vi "FPGAController_v3.vi"() -> ()   [LabVIEW 2012]
uses:
  <vilib>/Utility/miscctls.llb/LVPointTypeDef.ctl
  Functional Global Variables/Action Items.ctl
  <vilib>/FPGAPlugInAG/PXI-7954R/niLvFpga_Open_PXI-7954R.vi
  <vilib>/addons/database/Connection.llb/Conn Execute.vi
  <vilib>/addons/database/Recordset.llb/Rec Fetch Recordset Data (R).vi
  <vilib>/addons/database/Recordset.llb/Rec Destroy - Connection.vi
  <vilib>/Utility/error.llb/Error Cluster From Error Code.vi
  <vilib>/rvi/errors/niLvFpgaAdjustHostInterfaceError.vi
  <vilib>/FPGAPlugInAG/PXI-7954R/niLvFpga_Close_PXI-7954R.vi
  <vilib>/rvi/interface/nirviOpenFPGA/nirviOpenFPGA.xnode
  FPGA Bitfiles/correlationwithf_FPGATarget_ver1(FPGA)214201_xVEwbWkwy+w.lvbitx
  ver1(FPGA)_7_8_2013.vi
  <vilib>/rvi/interface/nirviMethod/nirviMethod.xnode
  <vilib>/FPGA/interface/niFpgaViExecutionMode.ctl
  <vilib>/addons/database/_DB Variant To Data/Database Variant To Data.xnode
  <vilib>/rvi/interface/nirviReadWriteControl/nirviReadWriteControl.xnode
  FPGA Bitfiles/correlationwithf_FPGATarget_ver1(FPGA)214201_RJg2enFNf9w.lvbitx
  <vilib>/rvi/interface/nirviCloseFPGA/nirviCloseFPGA.xnode
  <vilib>/addons/database/NI_Database_API.lvlib
  NiFpgaLv.dll
  <vilib>/FPGAPlugInAG/PXI-7954R/niLvFpga_Reset_PXI-7954R.vi
  <vilib>/FPGAPlugInAG/PXI-7954R/niLvFpga_Run_PXI-7954R.vi
panel:
  out "Rearm Trigger":bool
  in  "Rearm Trigger":bool
  in  "One Shot Mode":bool
  out "Last Update:":timestamp
  out "Updating FPGA":bool
  out "Sensitivity":dbl
  out "error out":errorcluster
  out "Low Mass Limit":fxp<+,31,17>
  out "High Mass Limit":fxp<+,31,17>
  out "stopping":bool
  in  "Auto Threshold":bool
  out "Peletron (MV)":dbl=2.0
  out "High Mass (kg)":dbl=inf
  out "Low Mass (kg)":dbl
  out "High Charge Limit":i16
  out "Low Charge Limit":i16
  out "High velocity count":i32=210
  out "Low velocity count":i32=21000
  in  "stop":bool
  in  "Peak-Threshold Factor":dbl=3.0
  out "Low Charge Limit (fC)":dbl
  out "High Charge Limit (fC)":dbl=100.0
  out "High Velocity":dbl=100000.0
  out "Low Velocity":dbl=1000.0
  out "Filter 7 Peak":i32=7483
  out "Filter 6 Peak":i32=9863
  out "Filter 5 Peak":i32=13910
  out "Filter 4 Peak":i32=18191
  out "Filter 3 Peak":i32=46254
  out "Filter 2 Peak":i32=120664
  out "Filter 1 Peak":i32=295996
  in  "Filter7 Threshold":i32=-21165
  in  "Filter6 Threshold":i32=-29358
  in  "Filter5 Threshold":i32=-41730
  in  "Filter4 Threshold":i32=-54306
  in  "Filter3 Threshold":i32=-138762
  in  "Filter2 Threshold":i32=-361992
  in  "Filter1 Threshold":i32=-887988
  in  "Zero Peak Values":bool
  in  "Assign Threshold":bool
  in  "Run Mode":bool
  # "Settings"
  # "Dubugging"
  # "Independent Variable"
  # "Low Vel."
  # "High Vel."
  # "Low Q (fC)"
  # "High Q (fC)"
  # "Plate Control While Loop Counter"
  # "Low Mass (kg)"
  # "High Mass (kg)"
  # "Sens. (V/pC)"
  # "Peletron (MV)"
  # "Current Value of Running Average"
  # "Peak Threshold Factor"
  # "Peak Values"
  # "Peak 1"
  # "Peak 2"
  # "Peak 3"
  # "Peak 4"
  # "Peak 5"
  # "Peak 6"
  # "Peak 7"
  # "Thresholds"
  # "Threshold 1"
  # "Threshold 2"
  # "Threshold 3"
  # "Threshold 4"
  # "Threshold 5"
  # "Threshold 6"
  # "Threshold 7"
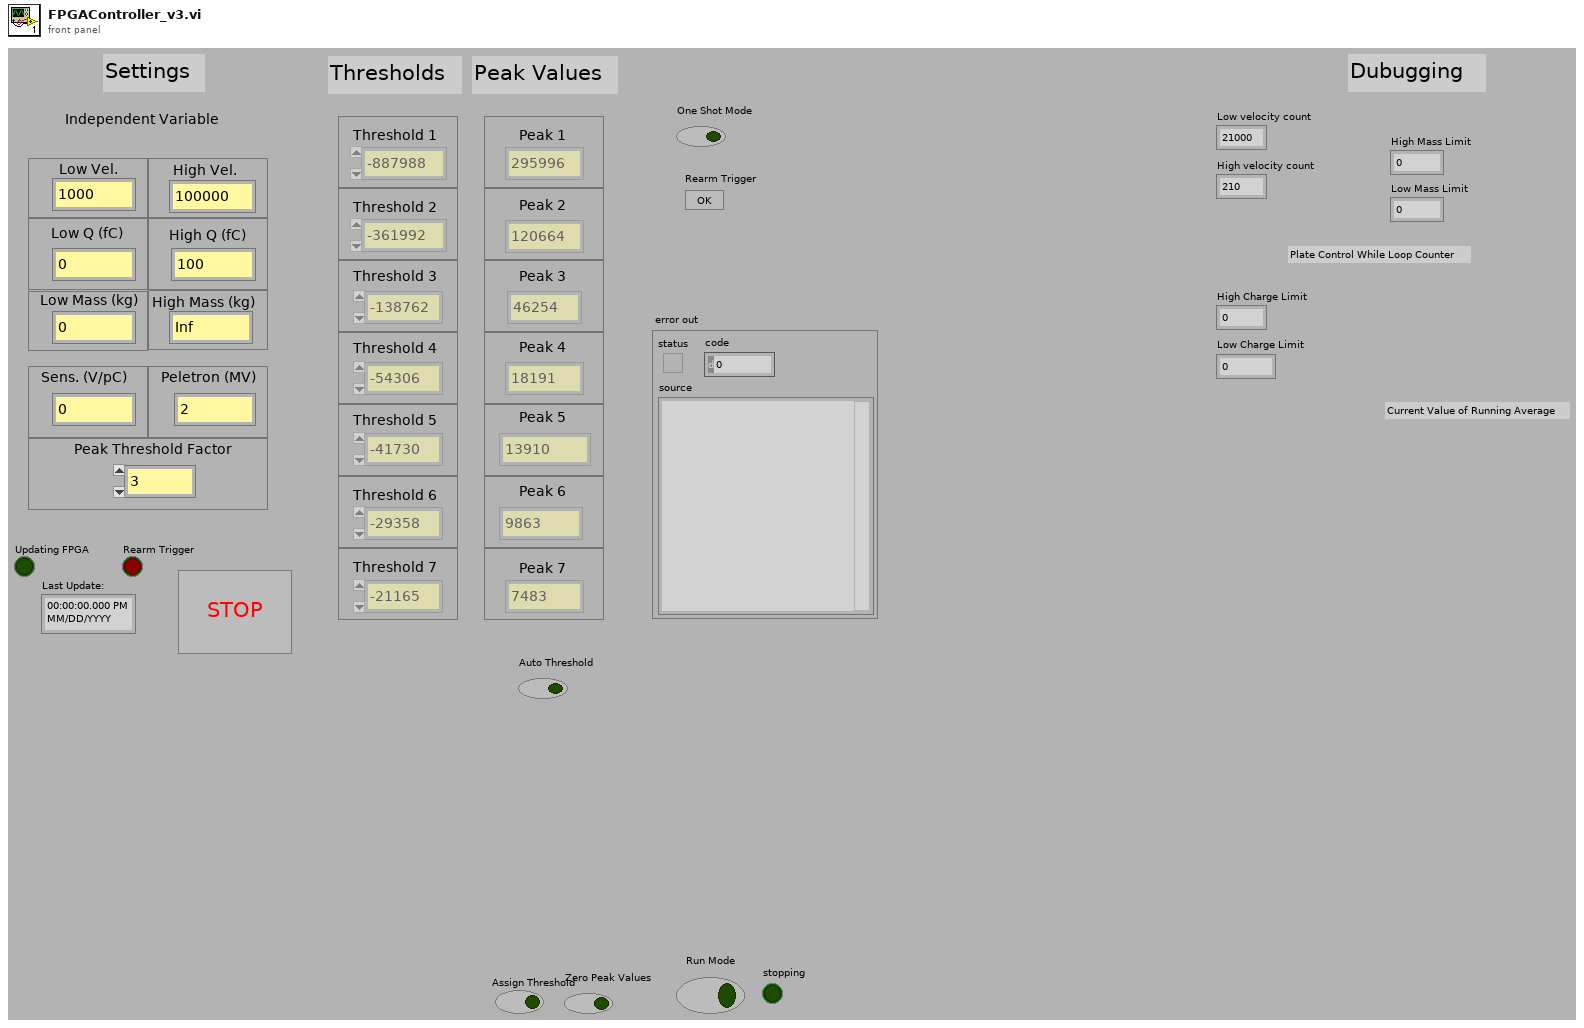
[diagram p1: front panel]
types:
  T1 = typedef "LVPointTypeDef.ctl" = cluster{"Horizontal":i16, "Vertical":i16}
  T2 = enum8{"Enabled", "Disabled", "Disabled and Grayed Out"}
  T3 = typedef "NI_Database_API.lvlib/Conn ObjectReference.ctl" = refnum<k1>
  T4 = typedef "Action Items.ctl" = enum16{"Initialize", "Get", "Set"}
  T5 = cluster{"Filter 1 Peak":i32, "Filter 2 Peak":i32, "Filter 3 Peak":i32, "Filter 4 Peak":i32, "Filter 5 Peak":i32, "Filter 6 Peak":i32, "Filter 7 Peak":i32}
  T6 = typedef "NI_Database_API.lvlib/Rec ObjectReference.ctl" = refnum<k1>
  T7 = cluster{"Numeric":dbl, "Numeric":dbl, "Numeric":dbl, "Numeric":dbl, "Numeric":dbl, "Numeric":dbl, dbl, dbl, "Value":dbl}
  T8 = cluster{"Low Velocity Count":i32, "High Velocity Count":i32, "Low Charge Limit (ADC ticks)":i16, "High Charge Limit (ADC ticks)":i16, "Low Mass (ADC*cycle^2)":i64, "High Mass (ADC*cycle^2)":i64}
  T9 = cluster{"Filter 1 Detector 3 Correlation":i32, "Filter 2 Detector 3 Correlation":i32, "Filter 3 Detector 3 Correlation":i32, "Filter 4 Detector 3 Correlation":i32, "Filter 5 Detector 3 Correlation":i32, "Filter 6 Detector 3 Correlation":i32, "Filter 7 Detector 3 Correlation":i32}
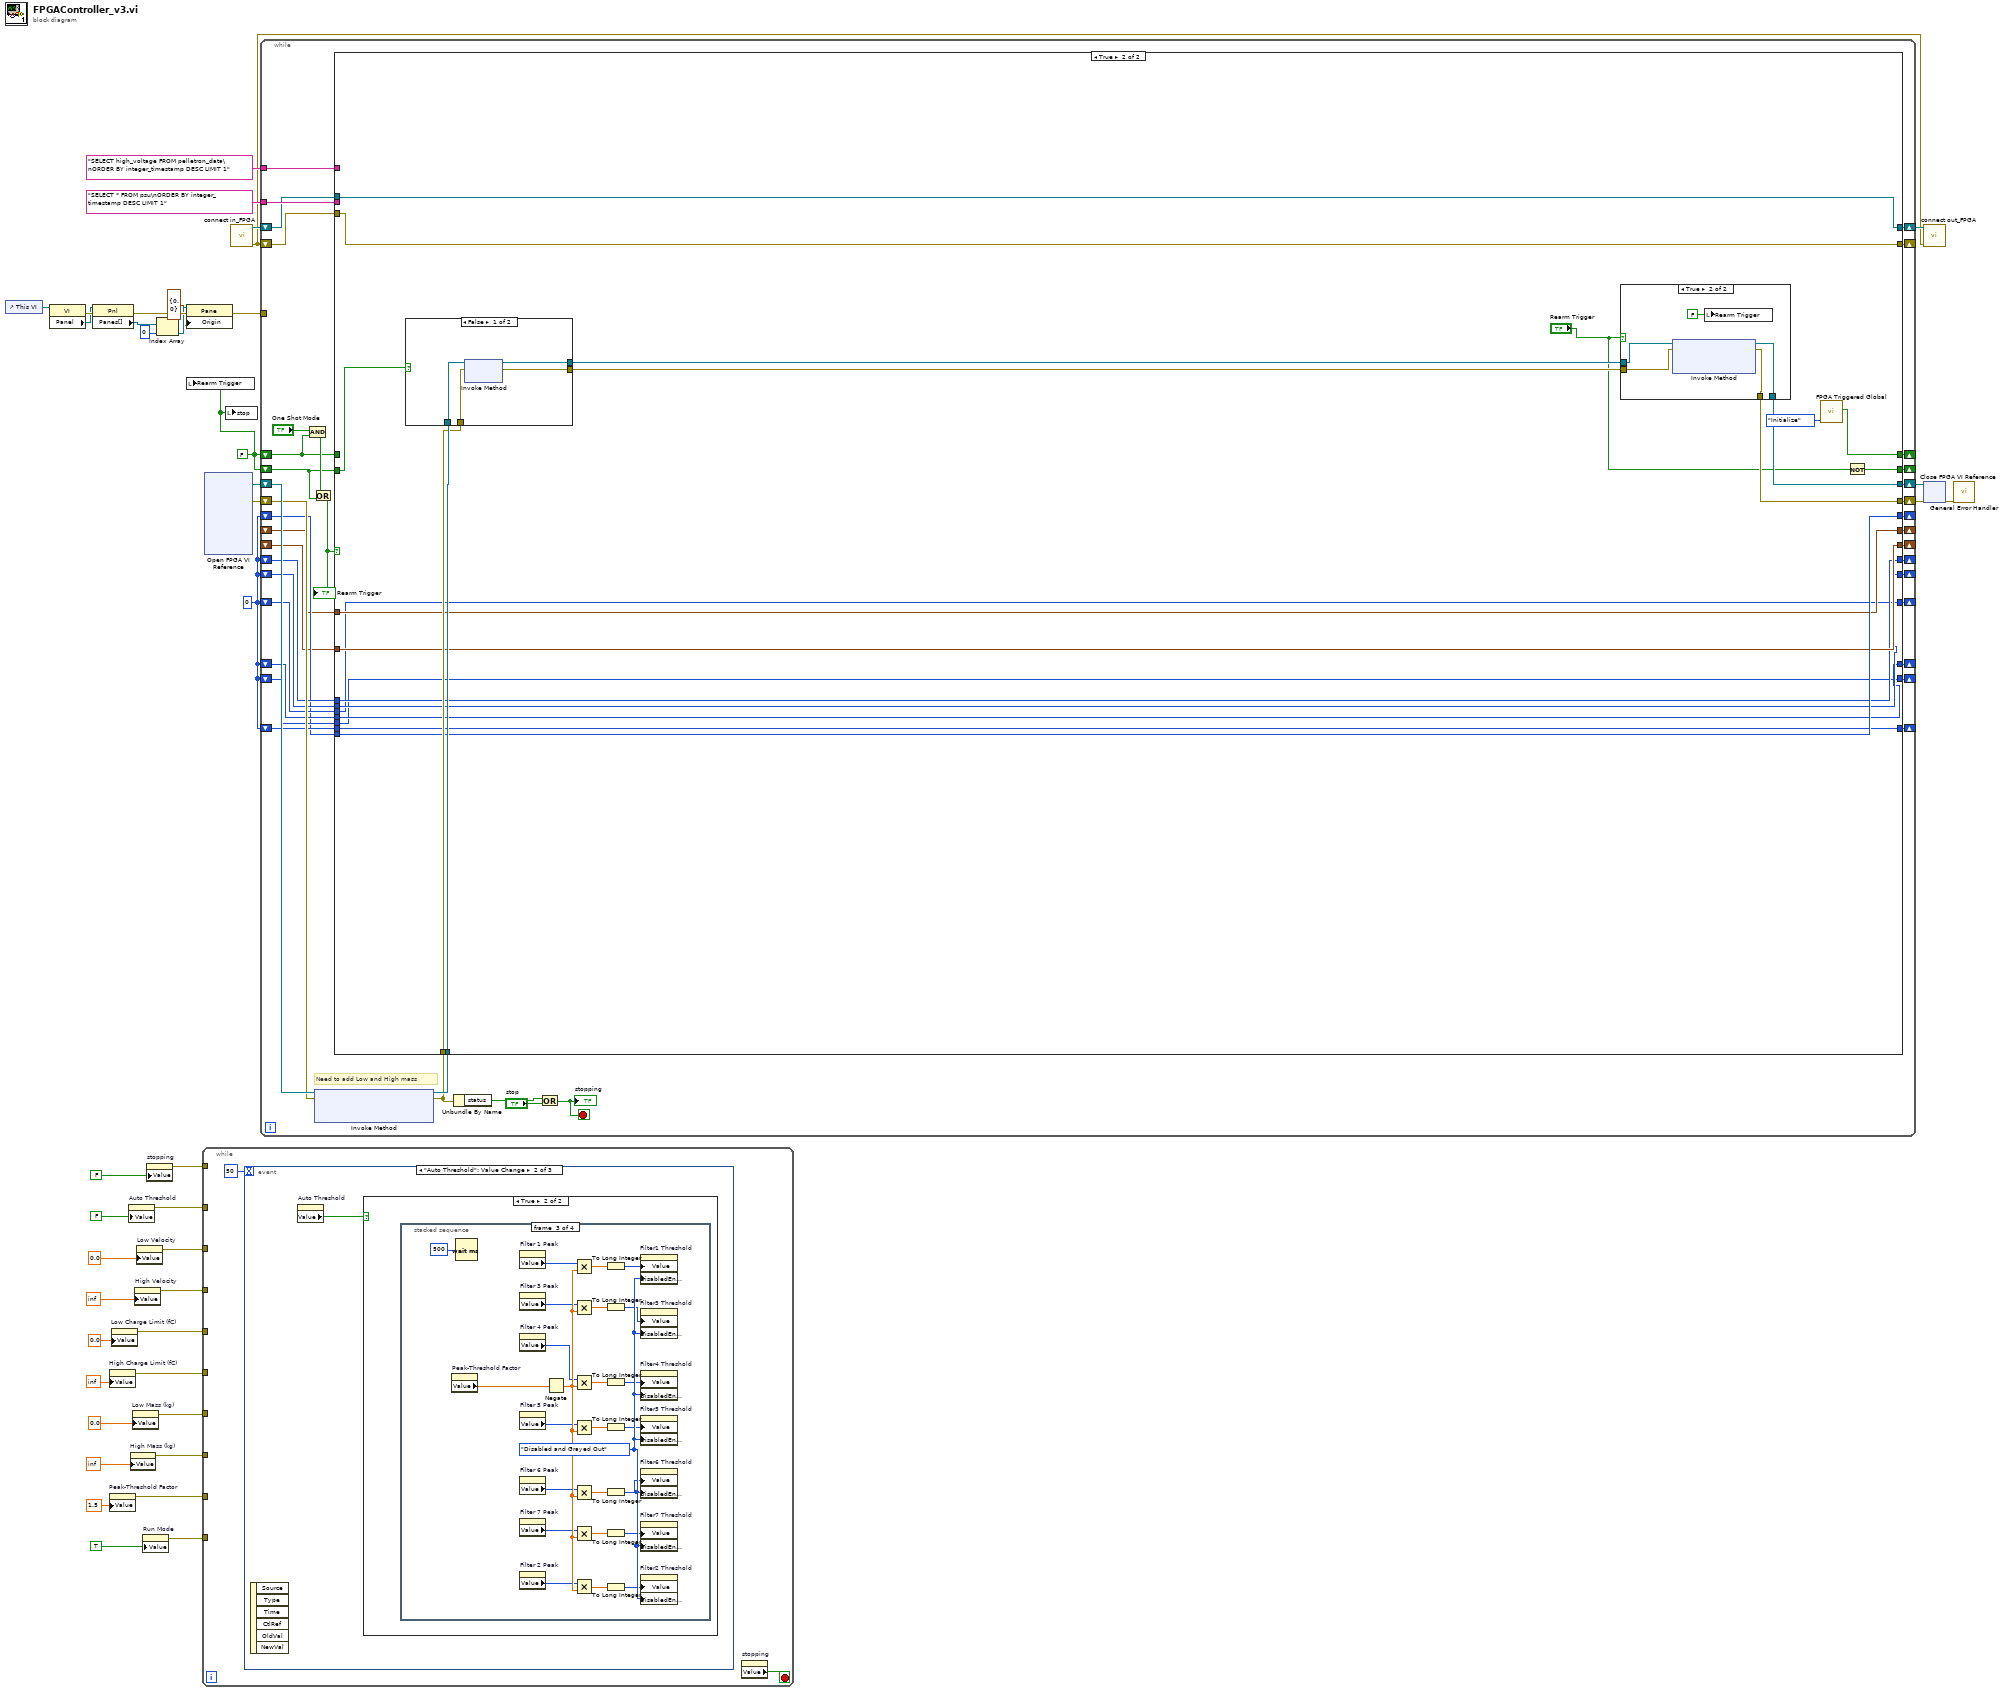
[diagram p0: block diagram]
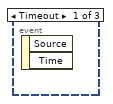
[diagram p2: hidden frame]
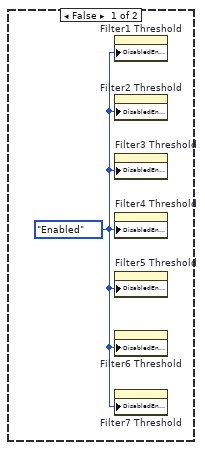
[diagram p3: hidden frame]
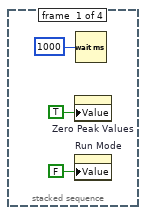
[diagram p4: hidden frame]
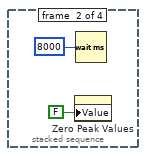
[diagram p5: hidden frame]
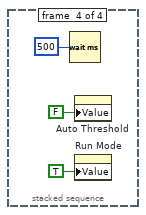
[diagram p6: hidden frame]
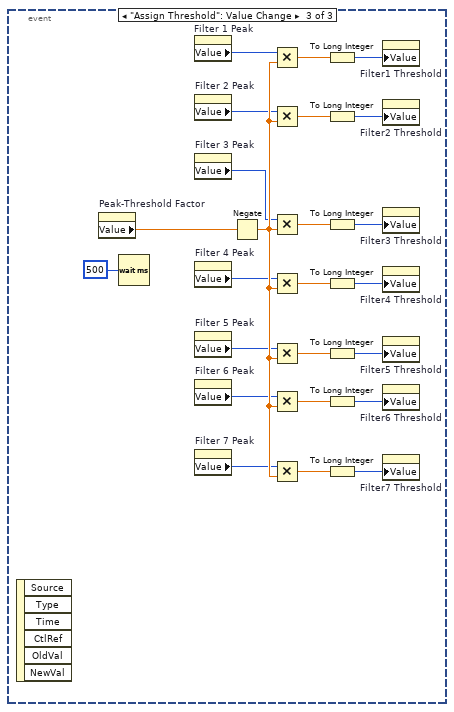
[diagram p7: hidden frame]
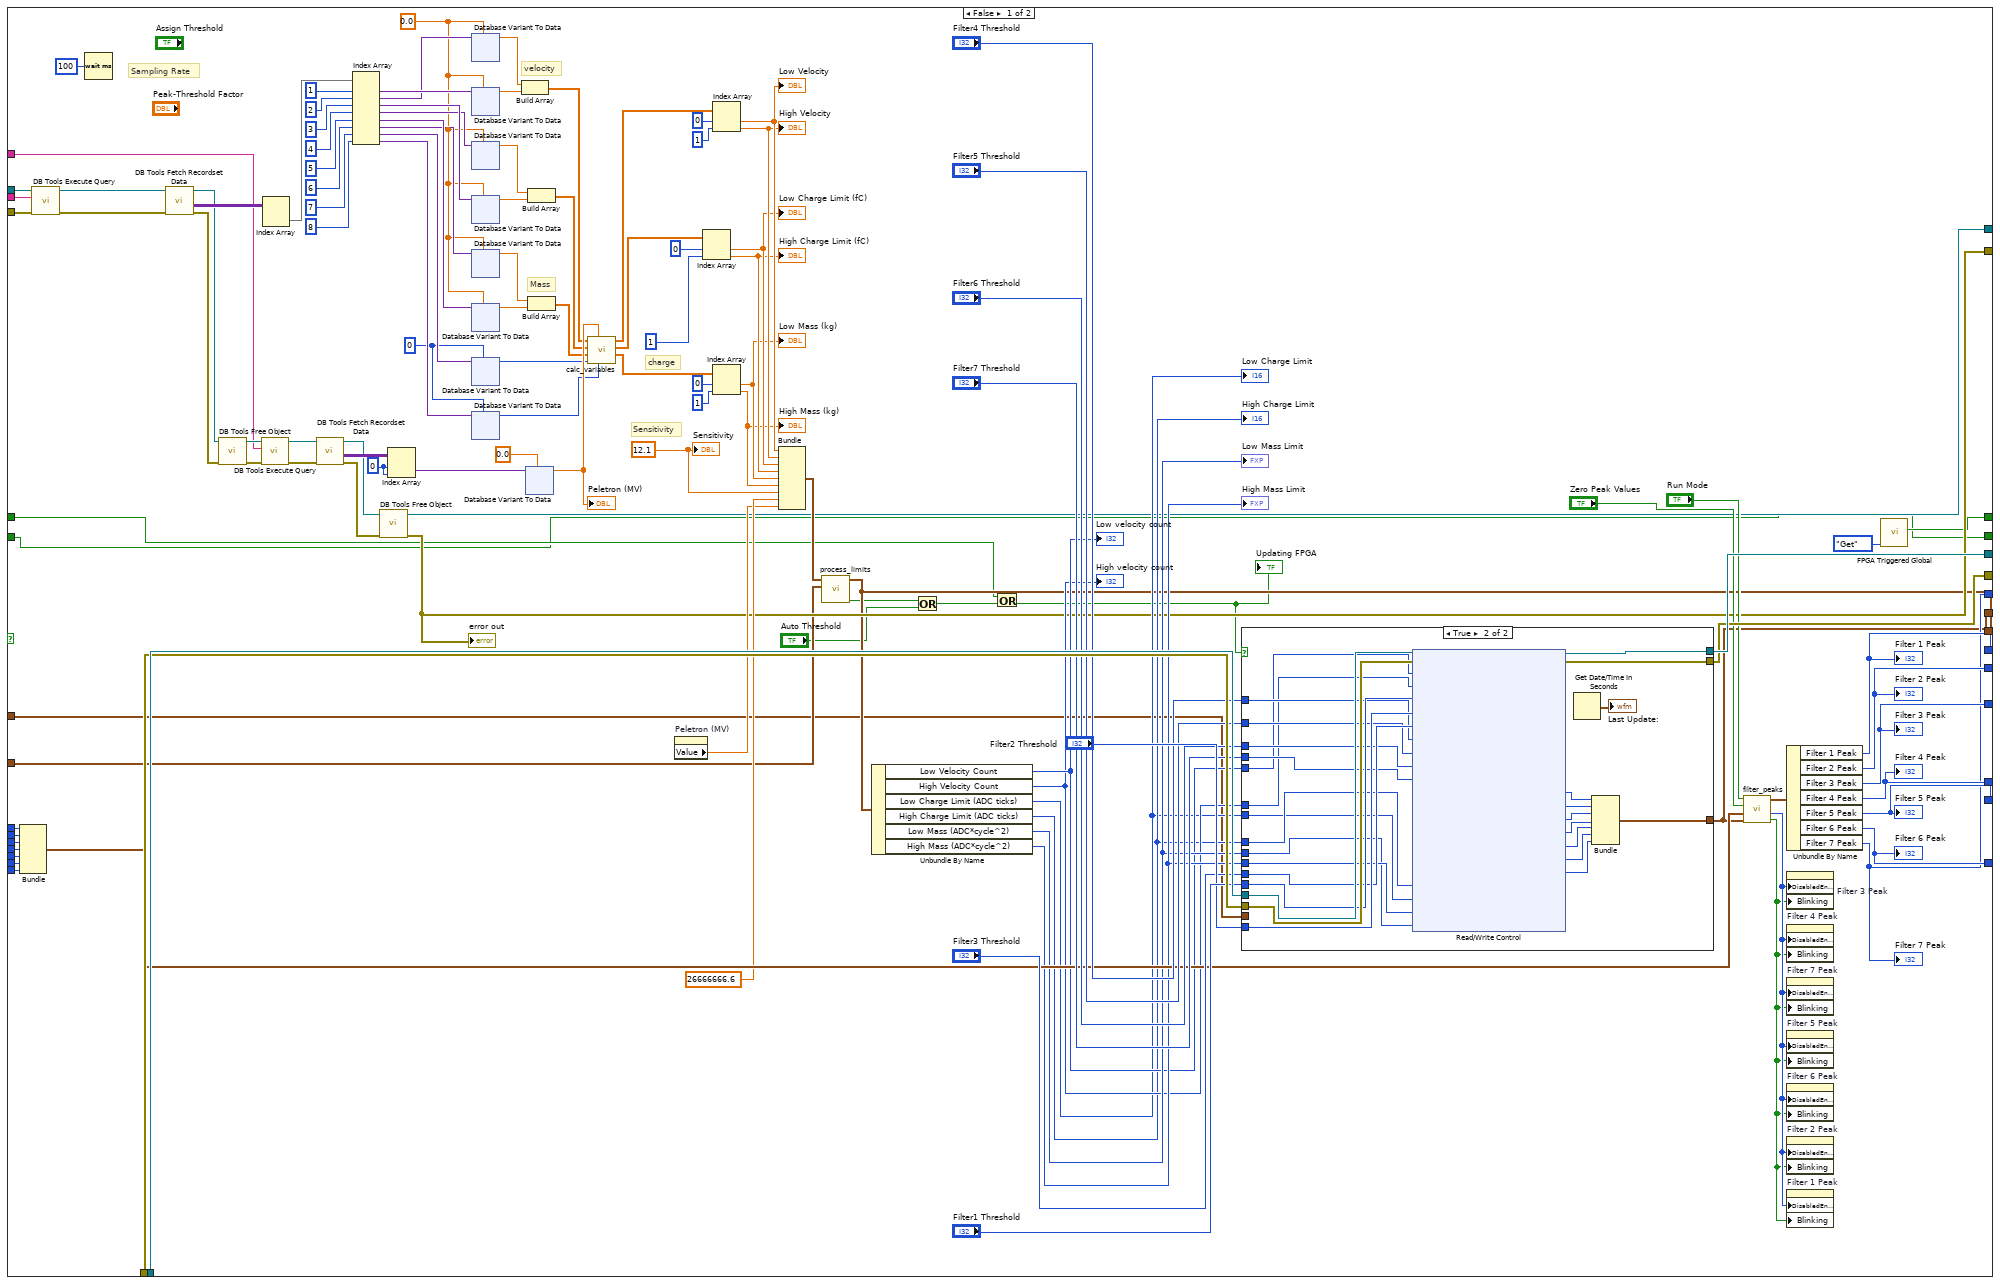
[diagram p8: hidden frame]
diagram:
  w1 = FALSE
  w40 = 0
  n1 = control-ref of="This VI"() -> (w10:refnum<vi>)
  n2 = property class="VI"(reference=w10) -> (error out=w9:errorcluster, "Panel"=w8:refnum<vi>)  [unwired: 1 in, 1 out]
  n3 = property class="Pnl"(reference=w8, error in=w9) -> (error out=w7:errorcluster, "Panes[]"=w6:refnum<vi>[])  [unwired: 1 out]
  n4 = property on="High Charge Limit (fC)" class="DigNum (strict)"("Value"=inf ("High Charge Limit (fC)")) -> (error out=w25:errorcluster)  [unwired: 2 in, 1 out]
  n5 = property on="Peak-Threshold Factor" class="DigNum (strict)"("Value"=1.5 ("Peak-Threshold Factor")) -> (error out=w19:errorcluster)  [unwired: 2 in, 1 out]
  n6 = property on="Low Charge Limit (fC)" class="DigNum (strict)"("Value"=0.0 ("Low Charge Limit (fC)")) -> (error out=w27:errorcluster)  [unwired: 2 in, 1 out]
  n7 = property on="Auto Threshold" class="Bool (strict)"("Value"=FALSE ("Auto Threshold")) -> (error out=w33:errorcluster)  [unwired: 2 in, 1 out]
  n8 = property on="High Mass (kg)" class="DigNum (strict)"("Value"=inf ("High Mass (kg)")) -> (error out=w21:errorcluster)  [unwired: 2 in, 1 out]
  n9 = property on="Low Mass (kg)" class="DigNum (strict)"("Value"=0.0 ("Low Mass (kg)")) -> (error out=w23:errorcluster)  [unwired: 2 in, 1 out]
  n10 = property on="High Velocity" class="DigNum (strict)"("Value"=inf ("High Velocity")) -> (error out=w29:errorcluster)  [unwired: 2 in, 1 out]
  n11 = property on="Low Velocity" class="DigNum (strict)"("Value"=0.0 ("Low Velocity")) -> (error out=w31:errorcluster)  [unwired: 2 in, 1 out]
  n12 = property on="Run Mode" class="Bool (strict)"("Value"=TRUE ("Run Mode")) -> (error out=w17:errorcluster)  [unwired: 2 in, 1 out]
  n13 = property on="stopping" class="Bool (strict)"("Value"=FALSE ("stopping")) -> (error out=w35:errorcluster)  [unwired: 2 in, 1 out]
  n14 = Index Array(array=w6, index=0) -> (element=w4:refnum<vi>)
  n15 = property class="Pane"(reference=w4, error in=w7, "Origin"=T1 {"Horizontal"=0, "Vertical"=0}) -> (error out=w2:errorcluster)  [unwired: 1 out]
  n16 = local write "Rearm Trigger"(w1) -> ()
  n17 = while {
    tunnel: w35 -> [_]
    tunnel: w33 -> [_]
    tunnel: w31 -> [_]
    tunnel: w29 -> [_]
    tunnel: w27 -> [_]
    tunnel: w25 -> [_]
    tunnel: w23 -> [_]
    tunnel: w21 -> [_]
    tunnel: w19 -> [_]
    tunnel: w17 -> [_]
    stop <- w43 stop-if-true
    n18 = event shown="[1] \"Auto Threshold\": Value Change" {
      selector: _ -> [_ _ _]
      dyn-events: _ -> [_ _ _]
      timeout: 50 -> [_ _ _]
      event Timeout {
        n19 = event-data() -> ()  [unwired: 1 in, 2 out]
      }
      event "Auto Threshold": Value Change {
        n20 = event-data() -> ()  [unwired: 1 in, 6 out]
        n21 = property on="Auto Threshold" class="Bool (strict)"() -> ("Value"=w44:bool)  [unwired: 2 in, 2 out]
        n22 = case shown="True" w44 {
          frame False {
            w45 = T2."Enabled" ("Disabled")
            n23 = property on="Filter1 Threshold" class="DigNum (strict)"("DisabledEnum"=w45) -> ()  [unwired: 2 in, 2 out]
            n24 = property on="Filter2 Threshold" class="DigNum (strict)"("DisabledEnum"=w45) -> ()  [unwired: 2 in, 2 out]
            n25 = property on="Filter3 Threshold" class="DigNum (strict)"("DisabledEnum"=w45) -> ()  [unwired: 2 in, 2 out]
            n26 = property on="Filter4 Threshold" class="DigNum (strict)"("DisabledEnum"=w45) -> ()  [unwired: 2 in, 2 out]
            n27 = property on="Filter5 Threshold" class="DigNum (strict)"("DisabledEnum"=w45) -> ()  [unwired: 2 in, 2 out]
            n28 = property on="Filter6 Threshold" class="DigNum (strict)"("DisabledEnum"=w45) -> ()  [unwired: 2 in, 2 out]
            n29 = property on="Filter7 Threshold" class="DigNum (strict)"("DisabledEnum"=w45) -> ()  [unwired: 2 in, 2 out]
          }
          frame True {
            n30 = stacked-sequence {
              frame #0 {
                n31 = property on="Zero Peak Values" class="Bool (strict)"("Value"=TRUE ("Zero Peak Values")) -> ()  [unwired: 2 in, 2 out]
                n32 = property on="Run Mode" class="Bool (strict)"("Value"=FALSE ("Run Mode")) -> ()  [unwired: 2 in, 2 out]
                n33 = Wait (ms)(milliseconds to wait=u32 1000) -> ()  [unwired: 1 out]
              }
              frame #1 {
                n34 = property on="Zero Peak Values" class="Bool (strict)"("Value"=FALSE ("Zero Peak Values")) -> ()  [unwired: 2 in, 2 out]
                n35 = Wait (ms)(milliseconds to wait=u32 8000) -> ()  [unwired: 1 out]
              }
              frame #2 {
                w75 = T2."Disabled and Grayed Out" ("Disabled")
                n36 = property on="Peak-Threshold Factor" class="DigNum (strict)"() -> ("Value"=w60:dbl)  [unwired: 2 in, 2 out]
                n37 = Wait (ms)(milliseconds to wait=u32 500) -> ()  [unwired: 1 out]
                n38 = property on="Filter 1 Peak" class="DigNum (strict)"() -> ("Value"=w58:i32)  [unwired: 2 in, 2 out]
                n39 = property on="Filter 3 Peak" class="DigNum (strict)"() -> ("Value"=w56:i32)  [unwired: 2 in, 2 out]
                n40 = property on="Filter 4 Peak" class="DigNum (strict)"() -> ("Value"=w55:i32)  [unwired: 2 in, 2 out]
                n41 = property on="Filter 5 Peak" class="DigNum (strict)"() -> ("Value"=w54:i32)  [unwired: 2 in, 2 out]
                n42 = property on="Filter 6 Peak" class="DigNum (strict)"() -> ("Value"=w53:i32)  [unwired: 2 in, 2 out]
                n43 = property on="Filter 7 Peak" class="DigNum (strict)"() -> ("Value"=w52:i32)  [unwired: 2 in, 2 out]
                n44 = property on="Filter 2 Peak" class="DigNum (strict)"() -> ("Value"=w57:i32)  [unwired: 2 in, 2 out]
                n45 = Negate(x=w60) -> (-x=w59:dbl)
                n46 = Multiply(x=w58, y=w59) -> (x*y=w74:dbl)
                n47 = Multiply(x=w56, y=w59) -> (x*y=w70:dbl)
                n48 = Multiply(x=w55, y=w59) -> (x*y=w68:dbl)
                n49 = Multiply(x=w54, y=w59) -> (x*y=w66:dbl)
                n50 = Multiply(x=w53, y=w59) -> (x*y=w64:dbl)
                n51 = Multiply(x=w52, y=w59) -> (x*y=w62:dbl)
                n52 = Multiply(x=w57, y=w59) -> (x*y=w72:dbl)
                n53 = To Long Integer(number=w74) -> (32bit integer=w73:i32)
                n54 = To Long Integer(number=w70) -> (32bit integer=w69:i32)
                n55 = To Long Integer(number=w68) -> (32bit integer=w67:i32)
                n56 = To Long Integer(number=w66) -> (32bit integer=w65:i32)
                n57 = To Long Integer(number=w64) -> (32bit integer=w63:i32)
                n58 = To Long Integer(number=w62) -> (32bit integer=w61:i32)
                n59 = To Long Integer(number=w72) -> (32bit integer=w71:i32)
                n60 = property on="Filter1 Threshold" class="DigNum (strict)"("Value"=w73, "DisabledEnum"=w75) -> ()  [unwired: 2 in, 2 out]
                n61 = property on="Filter3 Threshold" class="DigNum (strict)"("Value"=w69, "DisabledEnum"=w75) -> ()  [unwired: 2 in, 2 out]
                n62 = property on="Filter4 Threshold" class="DigNum (strict)"("Value"=w67, "DisabledEnum"=w75) -> ()  [unwired: 2 in, 2 out]
                n63 = property on="Filter5 Threshold" class="DigNum (strict)"("Value"=w65, "DisabledEnum"=w75) -> ()  [unwired: 2 in, 2 out]
                n64 = property on="Filter6 Threshold" class="DigNum (strict)"("Value"=w63, "DisabledEnum"=w75) -> ()  [unwired: 2 in, 2 out]
                n65 = property on="Filter7 Threshold" class="DigNum (strict)"("Value"=w61, "DisabledEnum"=w75) -> ()  [unwired: 2 in, 2 out]
                n66 = property on="Filter2 Threshold" class="DigNum (strict)"("Value"=w71, "DisabledEnum"=w75) -> ()  [unwired: 2 in, 2 out]
              }
              frame #3 {
                n67 = Wait (ms)(milliseconds to wait=u32 500) -> ()  [unwired: 1 out]
                n68 = property on="Auto Threshold" class="Bool (strict)"("Value"=FALSE ("Auto Threshold")) -> ()  [unwired: 2 in, 2 out]
                n69 = property on="Run Mode" class="Bool (strict)"("Value"=TRUE ("Run Mode")) -> ()  [unwired: 2 in, 2 out]
              }
            }
          }
        }
      }
      event "Assign Threshold": Value Change {
        n70 = event-data() -> ()  [unwired: 1 in, 6 out]
        n71 = property on="Peak-Threshold Factor" class="DigNum (strict)"() -> ("Value"=w93:dbl)  [unwired: 2 in, 2 out]
        n72 = Wait (ms)(milliseconds to wait=u32 500) -> ()  [unwired: 1 out]
        n73 = property on="Filter 1 Peak" class="DigNum (strict)"() -> ("Value"=w92:i32)  [unwired: 2 in, 2 out]
        n74 = property on="Filter 2 Peak" class="DigNum (strict)"() -> ("Value"=w91:i32)  [unwired: 2 in, 2 out]
        n75 = property on="Filter 3 Peak" class="DigNum (strict)"() -> ("Value"=w90:i32)  [unwired: 2 in, 2 out]
        n76 = property on="Filter 4 Peak" class="DigNum (strict)"() -> ("Value"=w89:i32)  [unwired: 2 in, 2 out]
        n77 = property on="Filter 5 Peak" class="DigNum (strict)"() -> ("Value"=w88:i32)  [unwired: 2 in, 2 out]
        n78 = property on="Filter 6 Peak" class="DigNum (strict)"() -> ("Value"=w87:i32)  [unwired: 2 in, 2 out]
        n79 = property on="Filter 7 Peak" class="DigNum (strict)"() -> ("Value"=w86:i32)  [unwired: 2 in, 2 out]
        n80 = Negate(x=w93) -> (-x=w95:dbl)
        n81 = Multiply(x=w92, y=w95) -> (x*y=w102:dbl)
        n82 = Multiply(x=w91, y=w95) -> (x*y=w100:dbl)
        n83 = Multiply(x=w90, y=w95) -> (x*y=w99:dbl)
        n84 = Multiply(x=w89, y=w95) -> (x*y=w98:dbl)
        n85 = Multiply(x=w88, y=w95) -> (x*y=w97:dbl)
        n86 = Multiply(x=w87, y=w95) -> (x*y=w96:dbl)
        n87 = Multiply(x=w86, y=w95) -> (x*y=w101:dbl)
        n88 = To Long Integer(number=w102) -> (32bit integer=w85:i32)
        n89 = To Long Integer(number=w100) -> (32bit integer=w84:i32)
        n90 = To Long Integer(number=w99) -> (32bit integer=w83:i32)
        n91 = To Long Integer(number=w98) -> (32bit integer=w82:i32)
        n92 = To Long Integer(number=w97) -> (32bit integer=w81:i32)
        n93 = To Long Integer(number=w96) -> (32bit integer=w80:i32)
        n94 = To Long Integer(number=w101) -> (32bit integer=w79:i32)
        n95 = property on="Filter1 Threshold" class="DigNum (strict)"("Value"=w85) -> ()  [unwired: 2 in, 2 out]
        n96 = property on="Filter2 Threshold" class="DigNum (strict)"("Value"=w84) -> ()  [unwired: 2 in, 2 out]
        n97 = property on="Filter3 Threshold" class="DigNum (strict)"("Value"=w83) -> ()  [unwired: 2 in, 2 out]
        n98 = property on="Filter4 Threshold" class="DigNum (strict)"("Value"=w82) -> ()  [unwired: 2 in, 2 out]
        n99 = property on="Filter5 Threshold" class="DigNum (strict)"("Value"=w81) -> ()  [unwired: 2 in, 2 out]
        n100 = property on="Filter6 Threshold" class="DigNum (strict)"("Value"=w80) -> ()  [unwired: 2 in, 2 out]
        n101 = property on="Filter7 Threshold" class="DigNum (strict)"("Value"=w79) -> ()  [unwired: 2 in, 2 out]
      }
    }
    n102 = property on="stopping" class="Bool (strict)"() -> ("Value"=w43:bool)  [unwired: 2 in, 2 out]
  }
  n103 = xnode "Open FPGA VI Reference"() -> ("FPGA VI Reference Out"=w37:refnum<k20>, "error out"=w36:errorcluster)  [unwired: 2 in]
  n104 = local write "stop"(w1) -> ()
  n105 = call "connect in_FPGA.vi"() -> ("error out"=w11:errorcluster, "Database Connection"=w12:T3)  [unwired: 7 in, 1 out]
  n106 = while {
    shift-right: [w136] -> w39
    shift-left: w37 -> [w142]
    shift-right: [w135] -> w38
    shift-left: w36 -> [w141]
    shift-right: [w131] -> _
    shift-left: w40 -> [w124]
    shift-right: [w130] -> _
    shift-left: w40 -> [w123]
    shift-right: [w129] -> _
    shift-left: w40 -> [w122]
    shift-right: [w128] -> _
    shift-left: w40 -> [w121]
    shift-right: [w127] -> _
    shift-left: w40 -> [w120]
    shift-right: [w133] -> _
    shift-left: w40 -> [w126]
    shift-right: [w132] -> _
    shift-left: w40 -> [w125]
    tunnel: "SELECT * FROM psu\nORDER BY integer_timestamp DESC LIMIT 1" ("SQL query") -> [w119]
    tunnel: "SELECT high_voltage FROM pelletron_data\nORDER BY integer_timestamp DESC LIMIT 1" ("SQL query") -> [w118]
    shift-right: [w114] -> w13
    shift-left: w12 -> [w117]
    shift-right: [w115] -> _
    shift-left: w11 -> [w116]
    shift-right: [w113] -> _
    shift-left: _ -> [w112]
    shift-right: [w110] -> _
    shift-left: _ -> [w111]
    tunnel: w2 -> [_]
    shift-right: [w109] -> _
    shift-left: w1 -> [w107]
    shift-right: [w104] -> _
    shift-left: w1 -> [w105]
    stop <- w134 stop-if-true
    # "Need to add Low and High mass"
    n107 = And(x="One Shot Mode", y=w107) -> (x .and. y?=w108:bool)
    n108 = Or(x=w108, y=w105) -> (x .or. y?=w106:bool)
    "Rearm Trigger" <- w106
    n109 = xnode "Invoke Method"("FPGA VI Reference In"=w142, "error in"=w141) -> ("FPGA VI Reference Out"=w138:refnum<k20>, "error out"=w137:errorcluster)  [unwired: 1 out]
    n110 = case shown="True" w106 {
      tunnel: w138 -> [w263 w598]
      tunnel: w137 -> [w262 w597]
      tunnel: [w261 w596] -> w136
      tunnel: [w260 w593] -> w135
      tunnel: [w249 w587] -> w133
      tunnel: [w248 w586] -> w132
      tunnel: [w247 w585] -> w131
      tunnel: [w246 w584] -> w130
      tunnel: [w245 w583] -> w129
      tunnel: [w244 w582] -> w128
      tunnel: [w243 w590] -> w127
      tunnel: w126 -> [w242 w587]
      tunnel: w125 -> [w241 w586]
      tunnel: w124 -> [w240 w585]
      tunnel: w123 -> [w239 w584]
      tunnel: w122 -> [w238 w583]
      tunnel: w121 -> [w237 w582]
      tunnel: w120 -> [w236 w590]
      tunnel: w119 -> [w224 _]
      tunnel: w118 -> [w197 _]
      tunnel: w117 -> [w162 w602]
      tunnel: w116 -> [w161 w601]
      tunnel: [w158 w601] -> w115
      tunnel: [w157 w602] -> w114
      tunnel: [w155 w588] -> w113
      tunnel: w112 -> [w154 w588]
      tunnel: w111 -> [w150 w589]
      tunnel: [w149 w589] -> w110
      tunnel: w107 -> [w146 _]
      tunnel: [w145 w581] -> w109
      tunnel: w105 -> [w143 w599]
      tunnel: [w143 w591] -> w104
      frame False {
        w193 = 0 ("index (row)")
        w202 = i8 0
        w203 = 0.0
        w156 = 12.1
        # "Mass"
        # "charge"
        # "velocity"
        # "Sensitivity"
        # "Sampling Rate"
        n111 = Bundle("Filter 1 Peak"=w242, "Filter 2 Peak"=w241, "Filter 3 Peak"=w240, "Filter 4 Peak"=w239, "Filter 5 Peak"=w238, "Filter 6 Peak"=w237, "Filter 7 Peak"=w236) -> (w235:T5)  [unwired: 1 in]
        n112 = call-poly <vilib>:"DB Tools Execute Query.vi"("error in (no error)"=w161, "SQL query"=w224, "connection reference"=w162) -> ("error out"=w222:errorcluster, "recordset reference"=w223:T6)  [unwired: 5 in]
        n113 = Wait (ms)(milliseconds to wait=u32 100) -> ()  [unwired: 1 out]
        n114 = call-poly <vilib>:"DB Tools Fetch Recordset Data.vi"("error in (no error)"=w222, "recordset reference"=w223) -> ("error out"=w200:errorcluster, "recordset data"=w213:variant[][], "recordset reference out"=w201:T6)  [unwired: 3 in]
        n115 = call-poly <vilib>:"DB Tools Free Object.vi"("error in (no error)"=w200, "recordset reference"=w201) -> ("error out"=w198:errorcluster, "connection reference"=w199:T3)  [unwired: 8 in]
        n116 = call-poly <vilib>:"DB Tools Execute Query.vi"("error in (no error)"=w198, "SQL query"=w197, "connection reference"=w199) -> ("error out"=w195:errorcluster, "recordset reference"=w196:T6)  [unwired: 5 in]
        n117 = Index Array(array=w213) -> (element=w212:variant[])  [unwired: 2 in]
        n118 = call-poly <vilib>:"DB Tools Fetch Recordset Data.vi"("error in (no error)"=w195, "recordset reference"=w196) -> ("error out"=w159:errorcluster, "recordset data"=w194:variant[][], "recordset reference out"=w160:T6)  [unwired: 3 in]
        n119 = Index Array(array=w212, index #1=1 ("index"), index #2=2 ("index"), index #3=3 ("index"), index #4=4 ("index"), index #5=5 ("index"), index #6=6 ("index"), index #7=7 ("index"), index #8=8 ("index")) -> (element #1=w211:variant, element #2=w210:variant, element #3=w209:variant, element #4=w208:variant, element #5=w207:variant, element #6=w206:variant, element #7=w205:variant, element #8=w204:variant)
        n120 = call-poly <vilib>:"DB Tools Free Object.vi"("error in (no error)"=w159, "recordset reference"=w160) -> ("error out"=w158:errorcluster, "connection reference"=w157:T3)  [unwired: 8 in]
        "error out" <- w158
        n121 = Index Array(array=w194, index (row)=w193, index (col)=w193) -> (element=w192:variant)
        n122 = xnode "Database Variant To Data"("database variant"=w210, "type"=w203) -> ("data"=w189:dbl)  [unwired: 1 in, 1 out]
        n123 = xnode "Database Variant To Data"("database variant"=w211, "type"=w203) -> ("data"=w188:dbl)  [unwired: 1 in, 1 out]
        n124 = xnode "Database Variant To Data"("database variant"=w208, "type"=w203) -> ("data"=w187:dbl)  [unwired: 1 in, 1 out]
        n125 = xnode "Database Variant To Data"("database variant"=w209, "type"=w203) -> ("data"=w186:dbl)  [unwired: 1 in, 1 out]
        n126 = xnode "Database Variant To Data"("database variant"=w206, "type"=w203) -> ("data"=w185:dbl)  [unwired: 1 in, 1 out]
        n127 = xnode "Database Variant To Data"("database variant"=w207, "type"=w203) -> ("data"=w184:dbl)  [unwired: 1 in, 1 out]
        n128 = xnode "Database Variant To Data"("database variant"=w205, "type"=w202) -> ("data"=w179:i8)  [unwired: 1 in, 1 out]
        n129 = xnode "Database Variant To Data"("database variant"=w204, "type"=w202) -> ("data"=w178:i8)  [unwired: 1 in, 1 out]
        n130 = Build Array(w189, w188) -> (w182:dbl[])
        n131 = xnode "Database Variant To Data"("database variant"=w192, "type"=0.0) -> ("data"=w183:dbl)  [unwired: 1 in, 1 out]
        "Peletron (MV)" <- w183
        n132 = Build Array(w187, w186) -> (w181:dbl[])
        n133 = Build Array(w185, w184) -> (w180:dbl[])
        n134 = call "calc_variables.vi"("var2"=w178, "Peletron"=w183, "var1"=w179, "Mass"=w180, "Charge"=w181, "Velocity"=w182) -> ("Mass out"=w171:dbl[], "Charge out"=w174:dbl[], "Velocity out"=w177:dbl[])  [unwired: 3 in]
        n135 = property on="Peletron (MV)" class="DigNum (strict)"() -> ("Value"=w190:dbl)  [unwired: 2 in, 2 out]
        n136 = Index Array(array=w174, index #1=0 ("index"), index #2=1 ("index")) -> (element #1=w166:dbl, element #2=w165:dbl)
        "High Charge Limit (fC)" <- w165
        "Low Charge Limit (fC)" <- w166
        n137 = Index Array(array=w177, index #1=0 ("index"), index #2=1 ("index")) -> (element #1=w168:dbl, element #2=w167:dbl)
        "High Velocity" <- w167
        "Low Velocity" <- w168
        n138 = Index Array(array=w171, index #1=0 ("index"), index #2=1 ("index")) -> (element #1=w164:dbl, element #2=w163:dbl)
        "Low Mass (kg)" <- w164
        "High Mass (kg)" <- w163
        n139 = Bundle("Numeric"=w168, "Numeric"=w167, "Numeric"=w166, "Numeric"=w165, "Numeric"=w164, "Numeric"=w163, w156, 26666666.6, "Value"=w190) -> (w234:T7)  [unwired: 1 in]
        n140 = call "process_limits.vi"("old output cluster"=w154, "Input cluster"=w234) -> ("Update FPGA"=w151:bool, "output cluster"=w155:T8)  [unwired: 8 in]
        n141 = Unbundle By Name(w155) -> ("Low Velocity Count"=w230:i32, "High Velocity Count"=w229:i32, "Low Charge Limit (ADC ticks)"=w227:i16, "High Charge Limit (ADC ticks)"=w228:i16, "Low Mass (ADC*cycle^2)"=w232:i64, "High Mass (ADC*cycle^2)"=w233:i64)
        "Low velocity count" <- w230
        "High velocity count" <- w229
        "High Charge Limit" <- w228
        "Low Charge Limit" <- w227
        "High Mass Limit" <- w233
        "Low Mass Limit" <- w232
        n142 = Or(x=w151, y="Auto Threshold") -> (x .or. y?=w153:bool)
        n143 = Or(x=w146, y=w153) -> (x .or. y?=w147:bool)
        "Updating FPGA" <- w147
        n144 = case shown="True" w147 {
          tunnel: w263 -> [w265 w292]
          tunnel: w262 -> [w266 w291]
          tunnel: [w265 w290] -> w261
          tunnel: [w266 w289] -> w260
          tunnel: "Filter1 Threshold" -> [_ w288]
          tunnel: "Filter2 Threshold" -> [_ w287]
          tunnel: "Filter3 Threshold" -> [_ w286]
          tunnel: "Filter4 Threshold" -> [_ w285]
          tunnel: "Filter5 Threshold" -> [_ w284]
          tunnel: "Filter6 Threshold" -> [_ w283]
          tunnel: "Filter7 Threshold" -> [_ w282]
          tunnel: [w264 w268] -> w149
          tunnel: w233 -> [_ w274]
          tunnel: w232 -> [_ w273]
          tunnel: w230 -> [_ w272]
          tunnel: w229 -> [_ w271]
          tunnel: w228 -> [_ w270]
          tunnel: w227 -> [_ w269]
          tunnel: w150 -> [w264 _]
          frame False {
          }
          frame True {
            n145 = xnode "Read/Write Control"("FPGA VI Reference In"=w292, "error in"=w291, "Low Velocity Count"=w272, "High Velocity Count"=w271, "Filter 1 threshold"=w288, "Filter 2 threshold"=w287, "Filter 3 threshold"=w286, "Filter 4 threshold"=w285, "Filter 5 threshold"=w284, "Filter 6 threshold"=w283, "Filter 7 threshold"=w282, "High Charge Limit"=w270, "Low Charge Limit"=w269, "High Mass Limit"=w274, "Low Mass Limit"=w273) -> ("FPGA VI Reference Out"=w290:refnum<k20>, "error out"=w289:errorcluster, "Filter 1 Detector 3 Correlation"=w281:i32, "Filter 2 Detector 3 Correlation"=w280:i32, "Filter 3 Detector 3 Correlation"=w279:i32, "Filter 4 Detector 3 Correlation"=w278:i32, "Filter 5 Detector 3 Correlation"=w277:i32, "Filter 6 Detector 3 Correlation"=w276:i32, "Filter 7 Detector 3 Correlation"=w275:i32)
            n146 = Get Date/Time In Seconds() -> (seconds since 1Jan1904=→"Last Update:":timestamp)
            n147 = Bundle("Filter 1 Detector 3 Correlation"=w281, "Filter 2 Detector 3 Correlation"=w280, "Filter 3 Detector 3 Correlation"=w279, "Filter 4 Detector 3 Correlation"=w278, "Filter 5 Detector 3 Correlation"=w277, "Filter 6 Detector 3 Correlation"=w276, "Filter 7 Detector 3 Correlation"=w275) -> (w268:T9)  [unwired: 1 in]
          }
        }
        n148 = call "filter_peaks.vi"("Correlation cluster"=w149, "Filter peak cluster"=w235, "Zero out"="Zero Peak Values", "Run Mode"="Run Mode") -> ("Blinking"=w226:bool, "status"=w231:T2, "Filter peak output"=w250:T5)  [unwired: 5 in]
        n149 = Unbundle By Name(w250) -> ("Filter 1 Peak"=w249:i32, "Filter 2 Peak"=w248:i32, "Filter 3 Peak"=w247:i32, "Filter 4 Peak"=w246:i32, "Filter 5 Peak"=w245:i32, "Filter 6 Peak"=w244:i32, "Filter 7 Peak"=w243:i32)
        "Filter 1 Peak" <- w249
        "Filter 2 Peak" <- w248
        "Filter 3 Peak" <- w247
        "Filter 4 Peak" <- w246
        "Filter 5 Peak" <- w245
        "Filter 6 Peak" <- w244
        "Filter 7 Peak" <- w243
        n150 = property on="Filter 3 Peak" class="DigNum (strict)"("DisabledEnum"=w231, "Blinking"=w226) -> ()  [unwired: 2 in, 2 out]
        n151 = property on="Filter 4 Peak" class="DigNum (strict)"("DisabledEnum"=w231, "Blinking"=w226) -> ()  [unwired: 2 in, 2 out]
        n152 = property on="Filter 7 Peak" class="DigNum (strict)"("DisabledEnum"=w231, "Blinking"=w226) -> ()  [unwired: 2 in, 2 out]
        n153 = property on="Filter 5 Peak" class="DigNum (strict)"("DisabledEnum"=w231, "Blinking"=w226) -> ()  [unwired: 2 in, 2 out]
        n154 = property on="Filter 6 Peak" class="DigNum (strict)"("DisabledEnum"=w231, "Blinking"=w226) -> ()  [unwired: 2 in, 2 out]
        n155 = property on="Filter 2 Peak" class="DigNum (strict)"("DisabledEnum"=w231, "Blinking"=w226) -> ()  [unwired: 2 in, 2 out]
        n156 = property on="Filter 1 Peak" class="DigNum (strict)"("DisabledEnum"=w231, "Blinking"=w226) -> ()  [unwired: 2 in, 2 out]
        n157 = call "FPGA Triggered Global.vi"("Action"=Action_Items."Get") -> ("FPGA Triggered?"=w145:bool)  [unwired: 10 in]
        "Sensitivity" <- w156
      }
      frame True {
        n158 = case shown="False" w599 {
          tunnel: w598 -> [w606 w608]
          tunnel: [w605 w608] -> w595
          tunnel: w597 -> [w604 w607]
          tunnel: [w603 w607] -> w594
          frame False {
            n159 = xnode "Invoke Method"("FPGA VI Reference In"=w606, "error in"=w604) -> ("FPGA VI Reference Out"=w605:refnum<k20>, "error out"=w603:errorcluster)
          }
          frame True {
          }
        }
        n160 = case shown="True" "Rearm Trigger" {
          tunnel: w595 -> [w610 w615]
          tunnel: [w610 w614] -> w596
          tunnel: w594 -> [w609 w613]
          tunnel: [w609 w612] -> w593
          frame False {
          }
          frame True {
            n161 = xnode "Invoke Method"("FPGA VI Reference In"=w615, "error in"=w613) -> ("FPGA VI Reference Out"=w614:refnum<k20>, "error out"=w612:errorcluster)  [unwired: 1 in]
            n162 = local write "Rearm Trigger"(FALSE ("Rearm Trigger")) -> ()
          }
        }
        n163 = call "FPGA Triggered Global.vi"("Action"=Action_Items."Initialize") -> ("FPGA Triggered?"=w581:bool)  [unwired: 10 in]
        n164 = Not(x="Rearm Trigger") -> (.not. x?=w591:bool)
      }
    }
    n165 = Unbundle By Name(w137) -> ("status"=w140:bool)
    n166 = Or(x=w140, y="stop") -> (x .or. y?=w134:bool)
    "stopping" <- w134
  }
  n167 = call "connect out_FPGA.vi"("error in (no error)"=w11, "connection reference"=w13) -> ()  [unwired: 9 in, 1 out]
  n168 = xnode "Close FPGA VI Reference"("FPGA VI Reference In"=w39, "error in"=w38) -> ("error out"=w41:errorcluster)
  n169 = call <vilib>:"General Error Handler.vi"("error in (no error)"=w41) -> ()  [unwired: 10 in, 5 out]
